vi "Write Browse Button_Disabled.vi"(5 "Browse Button:Disabled":u8, 9 "Path in":refnum<class "Path.lvclass">) -> (3 "Path out":refnum<class "Path.lvclass">)   [LabVIEW 2014, in "Path.lvclass"]
uses:
  Path.lvclass
  Path.lvclass/Path.ctl
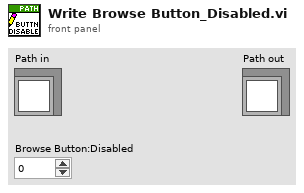
[diagram p1: front panel]
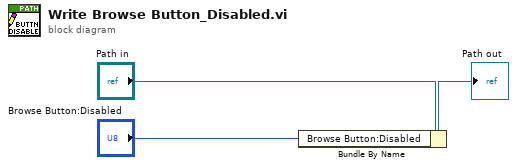
[diagram p0: block diagram]
diagram:
  n1 = Bundle By Name(cluster="Path in", "Browse Button:Disabled"="Browse Button:Disabled") -> (→"Path out":refnum<class "Path.lvclass">)
